vi "moveStage.vi"(1 "inc (mm)":dbl, 2 "axisIdx":i32=1, 3 "System no.":i32=1 min=1 max=4 step=1) -> (0 "Stopped":bool)   [LabVIEW 2015]
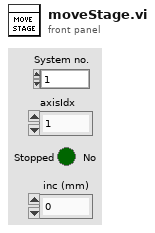
[diagram p1: front panel]
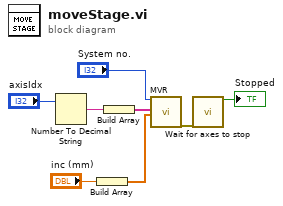
[diagram p0: block diagram]
diagram:
  n1 = Number To Decimal String(number="axisIdx") -> (decimal integer string=w5:string)  [unwired: 1 in]
  n2 = Build Array("inc (mm)") -> (w2:dbl[])
  n3 = Build Array(w5) -> (w3:string[])
  n4 = call "MVR.vi"("System no."="System no.", "Axes to move"=w3, "Position values"=w2) -> ("error out"=w8:errorcluster)  [unwired: 2 in, 14 out]
  n5 = call "Wait for axes to stop.vi"("error in"=w8) -> ("Stopped"=→"Stopped":bool)  [unwired: 6 in, 12 out]
